vi "USG_Query PAM.vi"(0 "System no.":i32=1 min=1 max=4 step=1, 2 "ContainerUnit":string, 3 "FunctionUnit":string, 4 "ParameterID":string, 5 "error in":errorcluster) -> (14 "Array of ParametersInfo":T1[](array[typedef]), 19 "error out":errorcluster)   [LabVIEW 2020]
doc: "USG? PAM (Parameter Overview)\n\nDescription\nOutputs the \"PAM\" section of the user guide.\nThe \"PAM\" section contains information on the parameters (p. 119) supported by the \ncontroller. Depending on the argument(s) used, the display is limited to certain parameters.\n\nFormat\nUSG? PAM[ <Container Unit>[ <Function Unit>[ <ParameterID>]]]\n\nArguments\n<Container Unit>\nContainer unit\nIf <Function Unit> and <ParameterID> are not specified, information about all parameters of \nthe container unit and the function units it contains are output.\nThe existing container units can be queried with USG? SYS.\nPossible values: Alias of the container unit (p. 94) \n<Function Unit>\nFunction unit\nIf <ParameterID> is not specified, information about all parameters of the function unit are \noutput.\nThe existing function units can be queried with USG? SYS.\nIf only information about the parameters that directly belong to the <Container Unit> is to be \noutput, \"-\" must be entered for <Function Unit>.\nPossible values:\nAlias of the function unit (p. 94) \n\"-\" \n<ParameterID>\n<ParameterID> always contains a parameter identifier in hexadecimal format. For 0-\ndimensional parameters, <ParameterID> is fully specified by the parameter identifier.\nFor one-dimensional and multi-dimensional parameters, an element address is also required \ntogether with the parameter identifier. Depending on the dimension of the parameter, the \nelement address consists of one or more parts that are separated from the parameter identifier \nand each other by a comma.\n- One-dimensional parameter (vector) ? the element address is ,number\n- Two-dimensional parameter (two-dimensional matrix) ? the element address is \n,number,number\n- Three-dimensional parameter (three-dimensional matrix) ? the element address \nis ,number,number,number\nThe address data for the parameters can be queried with USG? PAM (p. 77). \nPossible values:\n0x0000 to 0xFFFF\nFor one-dimensional and multi-dimensional parameters, an additional integer = 1 for each \ndimension\n\nResponse\nOnly the parameters that can be read in the current user command level (p. 69) are listed. The \noutput always has the following format:\nThe Parameter Overview section consists of at least the following fields:\n- Container Unit Alias (p. 94) for the container unit\n- Function Unit Alias (p. 94) for the function unit. The value \"-\" means that the parameter \nbelongs directly to the container unit.\n- Parameter ID Identifier of the parameter (p. 121) \n- Data Type Data type of the parameter, for details, see \"Permitted Data Types\" (p. 123). \n- Dimension Dimension of a parameter. The value \"-\" means that the parameter is 0-\ndimensional, i.e. it has exactly one value.\n- READ-UCL User command level, which is required at least to read the parameter. See \nUCL (p. 69) \n- WRITE-UCL User command level, which is required at least to write the parameter. See \nUCL (p. 69). The value \"-\" means that the parameter is write-protected (parameter of \ntype Unit Input, Unit Output and Unit Input-Output). \n- MINVALUE Minimum value of the parameter. The value \"-\" means that a minimum \nvalue is not sensible or necessary.\n- MAXVALUE Maximum value of the parameter. The value \"-\" means that a maximum \nvalue is not sensible or necessary.\n- Parameter Type Type of the parameter, for details, see \"Parameter Types\" (p. 119). \n- Description Description of the parameter.\nThe block can also have the following fields: \n- UNIT If the parameter has a unit, it is indicated here. Permitted characters: \"-\" (if no \nunits are given), \"phys. units\" (if the unit symbol for the parameter can be different, e.g. \nmm or µm), ??? defined unit symbols from measurement technology \n???(Warning)\"phys. units\" may only be used for one variable in the controller (normally \nthe control variable, e.g. the position).\n- Valid Values Possible values of the parameter. The value \"-\" means that specifying \npossible values is not sensible or necessary. If there are entries in this field, the \nparameter has the data type ENUM. For further details, see \"Permitted Data Types\"\n(p. 123). \n\nNotes\nUSG? without any arguments (p. 72) displays the contents of the user guide, i.e. the titles of the \navailable sections.\nUSG? PAM is comparable to HPA? or HPV? from GCS 2.0, but not identical to these commands.\n\nUser command level\nUSR"
uses:
  ParameterInfoSet.ctl
panel:
  # "USG? PAM (Parameter Overview)\n\nOutputs the \"PAM\" section of the user guide.\nThe \"PAM\" section contains information on the parameters supported by the controller. Depending on the argument(s) used, the display is limited to certain parameters."
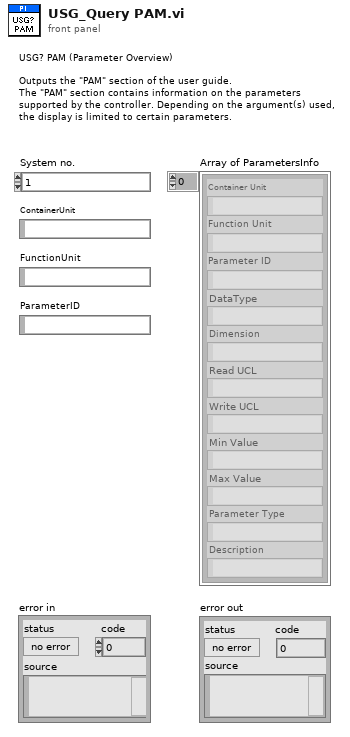
[diagram p1: front panel]
types:
  T1 = typedef "ParameterInfoSet.ctl" = cluster{"Container Unit":string, "Function Unit":string, "Parameter ID":string, "DataType":string, "Dimension":string, "Read UCL":string, "Write UCL":string, "Min Value":string, "Max Value":string, "Parameter Type":string, "Description":string}
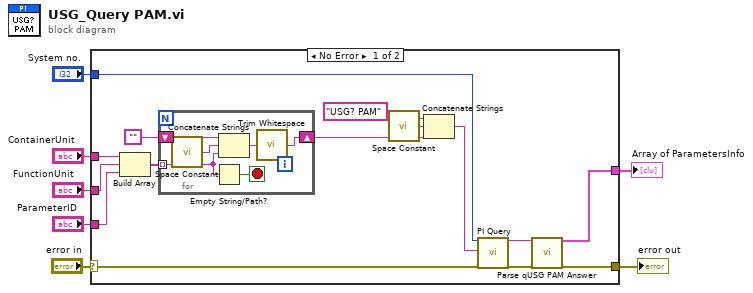
[diagram p0: block diagram]
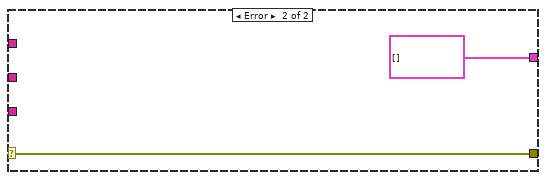
[diagram p2: hidden frame]
diagram:
  n1 = case shown="No Error" "error in" {
    selector: "error in" -> [w19 w30]
    tunnel: "System no." -> [w17 _]
    tunnel: [w9 w30] -> w6
    tunnel: "ContainerUnit" -> [w22 _]
    tunnel: "FunctionUnit" -> [w21 _]
    tunnel: "ParameterID" -> [w20 _]
    tunnel: [w8 T1[] [] ("Array of ParametersInfo")] -> w1
    frame No Error {
      n2 = Build Array(w22, w21, w20) -> (w12:string[])
      n3 = for {
        tunnel: w12 -> [w25] mode=indexing
        shift-right: [w27] -> w15
        shift-left: "" ("trimmed string") -> [w28]
        stop <- w23 stop-if-true
        n4 = call "Space Constant.vi"() -> ("String"=w26:string)
        n5 = Empty String/Path?(string/path=w25) -> (empty?=w23:bool)
        n6 = Concatenate Strings(w28, w26, w25) -> (w24:string)
        n7 = call "Trim Whitespace.vi"("string"=w24) -> ("trimmed string"=w27:string)  [unwired: 1 in]
      }
      n8 = call "Space Constant.vi"() -> ("String"=w14:string)
      n9 = Concatenate Strings("USG? PAM", w14, w15) -> (w18:string)
      n10 = call "PI Query.vi"("System no."=w17, "String to send"=w18, "error in"=w19) -> ("String read"=w11:string, "error out"=w10:errorcluster)  [unwired: 13 in, 2 out]
      n11 = call "Parse qUSG PAM Answer.vi"("Answer To Parse"=w11, "error in"=w10) -> ("Array of ParametersInfo"=w8:T1[], "error out"=w9:errorcluster)  [unwired: 16 in]
    }
    frame Error {
    }
  }
  "error out" <- w6
  "Array of ParametersInfo" <- w1
